vi "Save Initial Command.vi"(5 "Directory":string, 6 "Initial Path":dbl[][](array[numeric]), 7 "Path":path, 8 "z offset":dbl, 9 "y offset":dbl, 10 "x offset":dbl, 11 "form type":u16) -> (3 "Window Output":string)   [LabVIEW 2017]
uses:
  Globals.vi
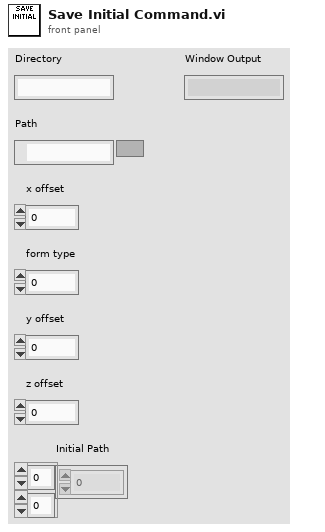
[diagram p1: front panel]
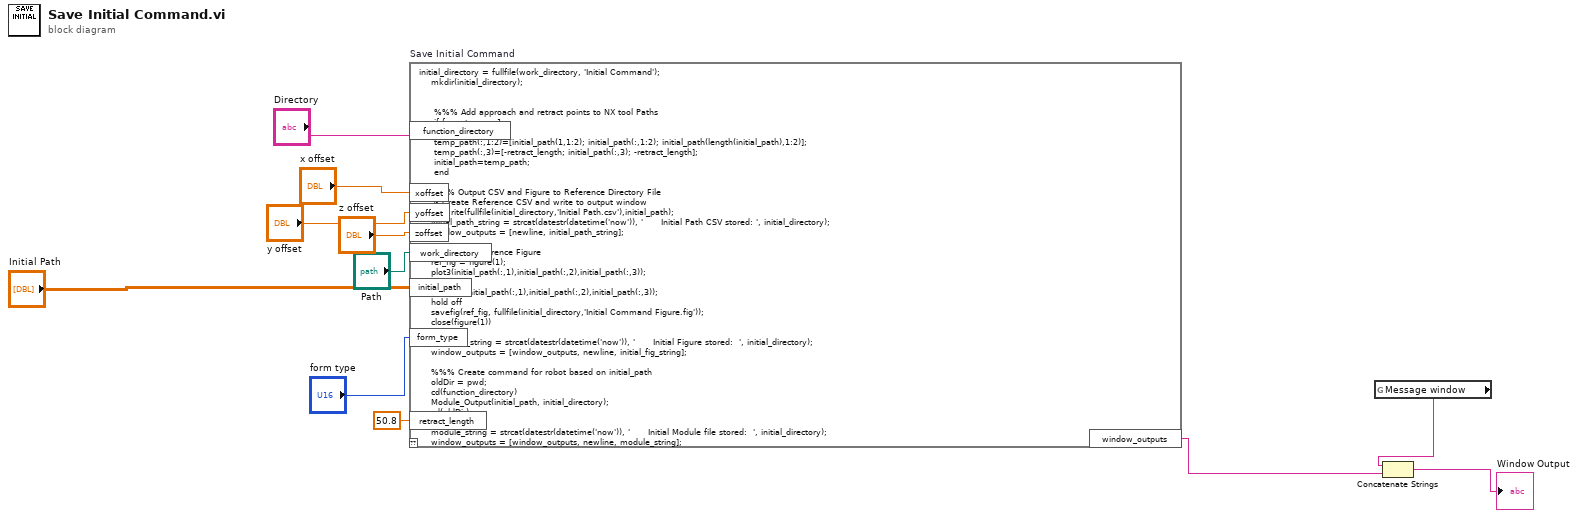
[diagram p0: block diagram]
diagram:
  n1 = script code="initial_directory = fullfile(work_directory, 'Initial Command');\n    mkdir(initial_directory);\n\n\n     %%% Add approach and retract points to NX tool Paths\n     if form_type==1\n     temp_path=[];\n     temp_path(:,1:2)=[initial_path(1,1:2); initial_path(:,1:2); initial_path(length(initial_path),1:2)];\n     temp_path(:,3)=[-retract_length; initial_path(:,3); -retract_length];\n     initial_path=temp_path;\n     end\n\n    %%% Output CSV and Figure to Reference Directory File\n    % Create Reference CSV and write to output window\n    csvwrite(fullfile(initial_directory,'Initial Path.csv'),initial_path);\n    initial_path_string = strcat(datestr(datetime('now')), '      Initial Path CSV stored: ', initial_directory);\n    window_outputs = [newline, initial_path_string];   \n\n    % Create Reference Figure    \n    ref_fig = figure(1);\n    plot3(initial_path(:,1),initial_path(:,2),initial_path(:,3));\n    hold on\n    scatter3(initial_path(:,1),initial_path(:,2),initial_path(:,3));\n    hold off\n    savefig(ref_fig, fullfile(initial_directory,'Initial Command Figure.fig'));\n    close(figure(1))\n\n    initial_fig_string = strcat(datestr(datetime('now')), '      Initial Figure stored:  ', initial_directory);\n    window_outputs = [window_outputs, newline, initial_fig_string];\n    \n    %%% Create command for robot based on initial_path\n    oldDir = pwd;\n    cd(function_directory)\n    Module_Output(initial_path, initial_directory);\n    cd(oldDir);\n\n    module_string = strcat(datestr(datetime('now')), '      Initial Module file stored:  ', initial_directory);\n    window_outputs = [window_outputs, newline, module_string];\n\n    % Print line divider to output window\n    window_outputs = [window_outputs, newline, ' ----------- ', newline];\n    \n\n        %%% Save inputs to work space\n        fileID = fopen(fullfile(initial_directory,'Initial Pyramid Parameters.txt'),'w');\n        fprintf(fileID,'Initial Parameters\\n');\n        fprintf(fileID,'X offset (mm): %4.3f\\n',xoffset);\n        fprintf(fileID,'Y offset (mm): %4.3f\\n',yoffset);\n        fprintf(fileID,'Z offset (mm): %4.3f\\n',zoffset);\n        fclose(fileID);" "Save Initial Command"("work_directory"="Path", "initial_path"="Initial Path", "form_type"="form type", "xoffset"="x offset", "yoffset"="y offset", "zoffset"="z offset", "function_directory"="Directory", "retract_length"=50.8 ("Real")) -> ("window_outputs"=w3:string)  [unwired: 1 in, 1 out]
  n2 = global read "Globals.vi" "Message window"() -> (w4:string)
  n3 = Concatenate Strings(w4, w3) -> (→"Window Output":string)
